vi "InitStreamTypeDef.vi"(9 "DAQ Node Array":string[](array[string]), 10 "DAQ Node Count":i32, 11 "StreamCluster_TypeDef":T1={"DAQ_Configs"=[], "CTR_Config"={"CTR refDes"="CTR001", "CTR IP Addr"="localhost"}, "Network_Configs"={"Buffer"=1, "ManagmentRate_Hz"=1000, "StreamRate_Hz"=10, "ConnectionHysterisis"=0, "LoggingRate_Hz"=10}, "ConfigXML_Checksum"=""}) -> (3 "StreamCluster_TypeDef":T1={"DAQ_Configs"=[], "CTR_Config"={"CTR refDes"="CTR001", "CTR IP Addr"="localhost"}, "Network_Configs"={"Buffer"=1, "ManagmentRate_Hz"=1000, "StreamRate_Hz"=10, "ConnectionHysterisis"=0, "LoggingRate_Hz"=10}, "ConfigXML_Checksum"=""})   [LabVIEW 2024]
uses:
  Control/StreamCluster_TypeDef.ctl
  Control/streamIO_states.ctl
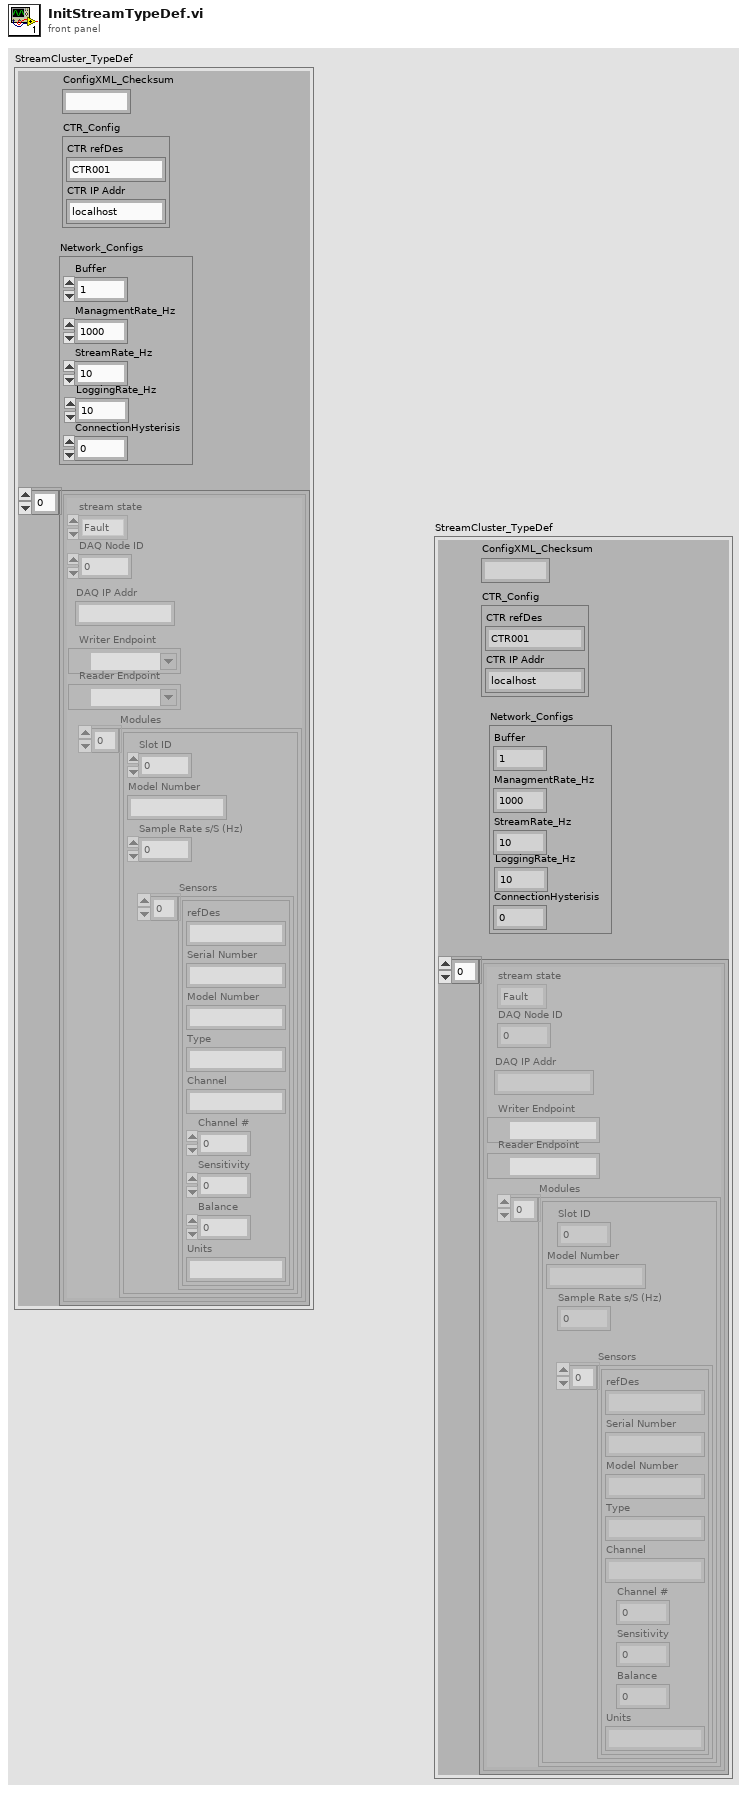
[diagram p1: front panel]
types:
  T1 = typedef "StreamCluster_TypeDef.ctl" = cluster{"DAQ_Configs":cluster{"stream state":T2, "DAQ Node ID":i32, "Writer Endpoint":refnum<k21>, "Reader Endpoint":refnum<k21>, "Modules":cluster{"Slot ID":i32, "Model Number":string, "Sample Rate s/S (Hz)":dbl, "Sensors":cluster{"refDes":string, "Serial Number":string, "Model Number":string, "Type":string, "Channel":string, "Channel #":i32, "Sensitivity":dbl, "Balance":dbl, "Units":string}[]}[], "DAQ IP Addr":string}[], "CTR_Config":cluster{"CTR refDes":string, "CTR IP Addr":string}, "Network_Configs":cluster{"Buffer":i32, "ManagmentRate_Hz":i32, "StreamRate_Hz":i32, "ConnectionHysterisis":i32, "LoggingRate_Hz":i32}, "ConfigXML_Checksum":string}
  T2 = typedef "streamIO_states.ctl" = enum16{"Fault", "Initialize", "Stream", "Close"}
  T3 = cluster{"stream state":T2, "DAQ Node ID":i32, "Writer Endpoint":refnum<k21>, "Reader Endpoint":refnum<k21>, "Modules":cluster{"Slot ID":i32, "Model Number":string, "Sample Rate s/S (Hz)":dbl, "Sensors":cluster{"refDes":string, "Serial Number":string, "Model Number":string, "Type":string, "Channel":string, "Channel #":i32, "Sensitivity":dbl, "Balance":dbl, "Units":string}[]}[], "DAQ IP Addr":string}[]
  T4 = cluster{"stream state":T2, "DAQ Node ID":i32, "Writer Endpoint":refnum<k21>, "Reader Endpoint":refnum<k21>, "Modules":cluster{"Slot ID":i32, "Model Number":string, "Sample Rate s/S (Hz)":dbl, "Sensors":cluster{"refDes":string, "Serial Number":string, "Model Number":string, "Type":string, "Channel":string, "Channel #":i32, "Sensitivity":dbl, "Balance":dbl, "Units":string}[]}[], "DAQ IP Addr":string}
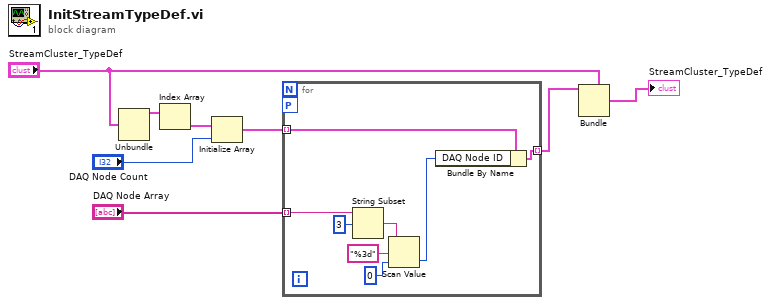
[diagram p0: block diagram]
diagram:
  n1 = Unbundle("StreamCluster_TypeDef") -> ("DAQ_Configs"=w4:T3)  [unwired: 3 out]
  n2 = Index Array(array=w4) -> (element=w8:T4)  [unwired: 1 in]
  n3 = Initialize Array(w8, "DAQ Node Count") -> (w5:T3)
  n4 = for {
    workers-P: _ -> [_]
    tunnel: "DAQ Node Array" -> [w12] mode=indexing
    tunnel: w5 -> [w9] mode=indexing
    tunnel: [w10] -> w3 mode=indexing
    n5 = String Subset(string=w12, offset (0)=3) -> (substring=w16:string)  [unwired: 1 in]
    n6 = Scan Value(string=w16, format string="%3d", default (0 dbl)=0) -> (value=w11:i32)  [unwired: 1 out]
    n7 = Bundle By Name(cluster=w9, "DAQ Node ID"=w11) -> (w10:T4)
  }
  n8 = Bundle(cluster="StreamCluster_TypeDef", "DAQ_Configs"=w3) -> (→"StreamCluster_TypeDef":T1)  [unwired: 3 in]
